vi "AO_control.vi"() -> ()   [LabVIEW 2020]
uses:
  <vilib>/DAQmx/write.llb/DAQmx Write (Analog 1D DBL NChan 1Samp).vi
  <vilib>/DAQmx/create/channels.llb/DAQmx Create Channel (AO-Voltage-Basic).vi
  <vilib>/DAQmx/miscellaneous.llb/DAQmx Fill In Error Info.vi
panel:
  in  "Power 561 nm (%)":dbl(slide) scale=0.0..100.0
  in  "stop":bool
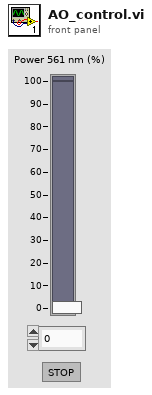
[diagram p1: front panel]
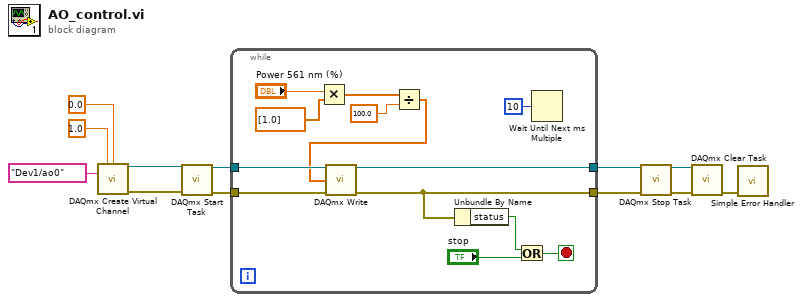
[diagram p0: block diagram]
diagram:
  n1 = call-poly <vilib>:"DAQmx Create Virtual Channel.vi"("maximum value"=1.0, "minimum value"=0.0, "physical channels"=tag "Dev1/ao0") -> ("task out"=w8:refnum<k21>, "error out"=w7:errorcluster)  [unwired: 11 in]
  n2 = call <vilib>:"DAQmx Start Task.vi"("task/channels in"=w8, "error in"=w7) -> ("task out"=w6:refnum<k21>, "error out"=w5:errorcluster)  [unwired: 12 in]
  n3 = while {
    tunnel: w6 -> [w24]
    tunnel: w5 -> [w23]
    tunnel: [w21] -> w4
    tunnel: [w20] -> w3
    stop <- w25 stop-if-true
    n4 = Multiply(x="Power 561 nm (%)", y=dbl[] [1.0] ("data")) -> (x*y=w16:dbl[])
    n5 = Divide(x=w16, y=100.0) -> (x/y=w15:dbl[])
    n6 = call-poly <vilib>:"DAQmx Write.vi"("task/channels in"=w24, "data"=w15, "error in"=w23) -> ("task out"=w20:refnum<k21>, "error out"=w21:errorcluster)  [unwired: 10 in, 1 out]
    n7 = Unbundle By Name(w21) -> ("status"=w22:bool)
    n8 = Or(x=w22, y="stop") -> (x .or. y?=w25:bool)
    n9 = Wait Until Next ms Multiple(millisecond multiple=u32 10) -> ()  [unwired: 1 out]
  }
  n10 = call <vilib>:"DAQmx Stop Task.vi"("task/channels in"=w3, "error in"=w4) -> ("task out"=w12:refnum<k21>, "error out"=w11:errorcluster)  [unwired: 12 in]
  n11 = call <vilib>:"DAQmx Clear Task.vi"("task in"=w12, "error in"=w11) -> ("error out"=w10:errorcluster)  [unwired: 13 in]
  n12 = call <vilib>:"Simple Error Handler.vi"("error in (no error)"=w10) -> ()  [unwired: 4 in, 5 out]
